vi "case_error.vi"() -> ()   [LabVIEW 2021]
panel:
  out "error out":errorcluster
  in  "error in (no error)":errorcluster
  out "Square Root":dbl
  in  "Square Root Input":dbl
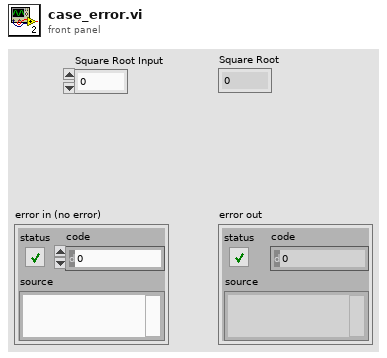
[diagram p1: front panel]
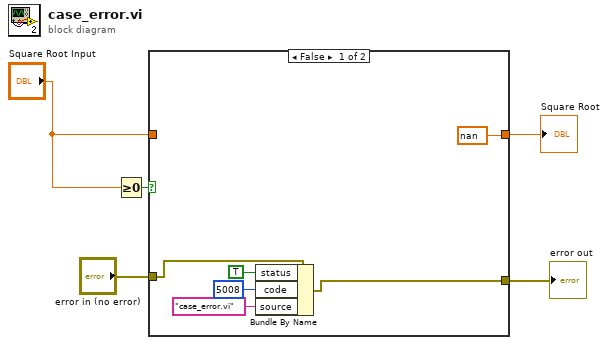
[diagram p0: block diagram]
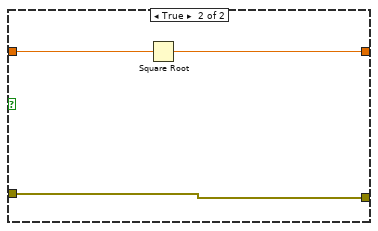
[diagram p2: hidden frame]
diagram:
  n1 = Greater Or Equal To 0?(x="Square Root Input") -> (x >= 0?=w5:bool)
  n2 = case shown="False" w5 {
    tunnel: [nan w14] -> w4
    tunnel: "Square Root Input" -> [_ w13]
    tunnel: [w6 w12] -> w2
    tunnel: "error in (no error)" -> [w10 w12]
    frame False {
      n3 = Bundle By Name(cluster=w10, "status"=TRUE, "code"=5008, "source"="case_error.vi") -> (w6:errorcluster)
    }
    frame True {
      n4 = Square Root(x=w13) -> (sqrt(x)=w14:dbl)
    }
  }
  "Square Root" <- w4
  "error out" <- w2
